vi "Trim Whitespace (String Array)__ogtk.vi"(5 "remove (leading and trailing)":enum16{"leading", "trailing", "both"}(ring)=enum."both", 6 "String in":string[](array[string])) -> (1 "String out":string[](array[string]))   [LabVIEW 2018]
doc: "Removes leading and/or trailing whitespace from a string.\nWhitespace is defined as any of the following characters (where values are in the format: dec, hex, string):\n <b>tab</b> = 9, 0x09, \\t\n <b>newline</b> = 10, 0x0A, \\n\n <b>vertical tab</b> = 11, 0x0B, \\0B\n <b>form feed</b> = 12, 0x0C, \\f\n <b>carriage return</b> = 13, 0x0D, \\r \n <b>space</b> = 32, 0x20, \\s\n\nThis VI is <b>reentrant</b>"
panel:
  # "Please visit http://www.OpenG.org to learn about the\nOpen Source LabVIEW software movement.\n\nNOTICE -- YOU MUST LEAVE THIS NOTICE IN PLACE.  PER THE TERMS OF THE LICENSE BELOW, YOU MAY SUBLICENSE THIS SOFTWARE \nIN ANY WAY THAT DOES NOT CONFLICT WITH THIS LICENSE.\n\n### BSD License (http://www.opensource.org/licenses/bsd-license.php) Begin ###\n \nCopyright (c) 2002-2006, Jim Kring <jim@jimkring.com>\nCopyright (c) 2002, Cal-Bay Systems, Inc. <info@calbay.com>\n\nAll rights reserved.\n\nRedistribution and use in source and binary forms, with or without modification, are permitted provided that the following conditions are met:\n\n    * Redistributions of source code must retain the above copyright notice, this list of conditions and the following disclaimer.\n    * Redistributions in binary form must reproduce the above copyright notice, this list of conditions and the following disclaimer in the \n       documentation and/or other materials provided with the distribution.\n    * Neither the name of SciWare, James Kring, Inc., nor the names of its contributors may be used to endorse or promote products derived \n       from this software without specific prior written permission.\n\nTHIS SOFTWARE IS PROVIDED BY THE COPYRIGHT HOLDERS AND CONTRIBUTORS \"AS IS\" AND ANY EXPRESS OR IMPLIED WARRANTIES, \nINCLUDING, BUT NOT LIMITED TO, THE IMPLIED WARRANTIES OF MERCHANTABILITY AND FITNESS FOR A PARTICULAR PURPOSE ARE \nDISCLAIMED. IN NO EVENT SHALL THE COPYRIGHT OWNER OR CONTRIBUTORS BE LIABLE FOR ANY DIRECT, INDIRECT, INCIDENTAL,\n SPECIAL, EXEMPLARY, OR CONSEQUENTIAL DAMAGES (INCLUDING, BUT NOT LIMITED TO, PROCUREMENT OF SUBSTITUTE GOODS OR \nSERVICES; LOSS OF USE, DATA, OR PROFITS; OR BUSINESS INTERRUPTION) HOWEVER CAUSED AND ON ANY THEORY OF LIABILITY, \nWHETHER IN CONTRACT, STRICT LIABILITY, OR TORT (INCLUDING NEGLIGENCE OR OTHERWISE) ARISING IN ANY WAY OUT OF THE USE \nOF THIS SOFTWARE, EVEN IF ADVISED OF THE POSSIBILITY OF SUCH DAMAGE.\n\n### BSD License End ###"
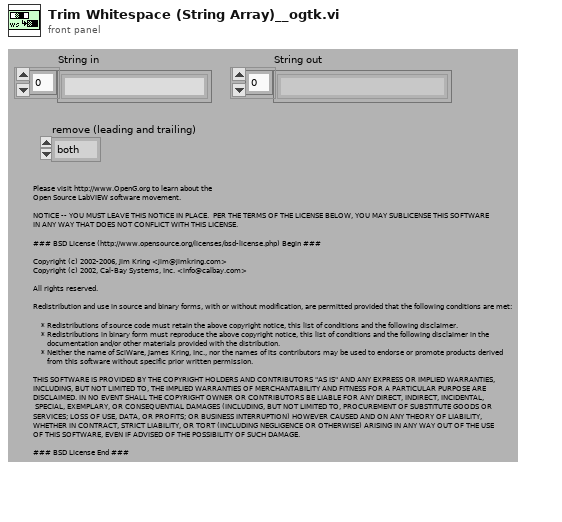
[diagram p1: front panel]
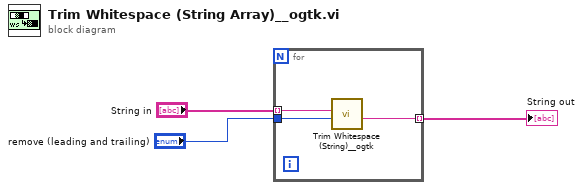
[diagram p0: block diagram]
diagram:
  n1 = for {
    tunnel: "remove (leading and trailing)" -> [w6]
    tunnel: "String in" -> [w5] mode=indexing
    tunnel: [w4] -> w1 mode=indexing
    n2 = call <userlib>:"Trim Whitespace (String)__ogtk.vi"("Remove (leading and trailing)"=w6, "String in"=w5) -> ("String out"=w4:string)  [unwired: 5 in]
  }
  "String out" <- w1
